vi "Testing (not part of comp).vi"() -> ()   [LabVIEW 2013]
panel:
  in  "Down":bool
  in  "Up":bool
  in  "ON/OFF":bool
  in  "Return":bool
  in  "stop":bool
  in  "4 ft":bool
  # "Pickup"
  # "LED"
  # "Shooter"
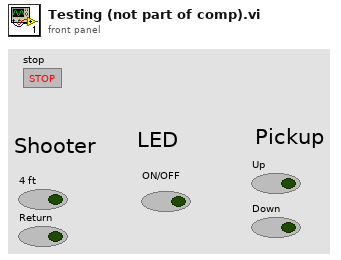
[diagram p1: front panel]
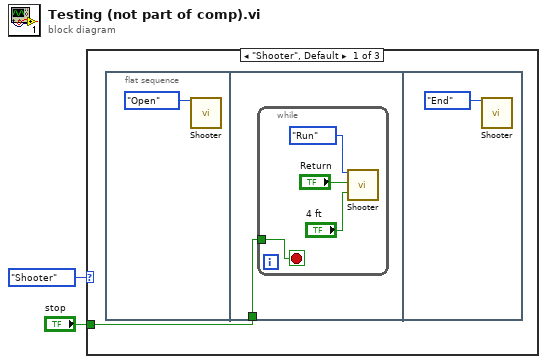
[diagram p0: block diagram]
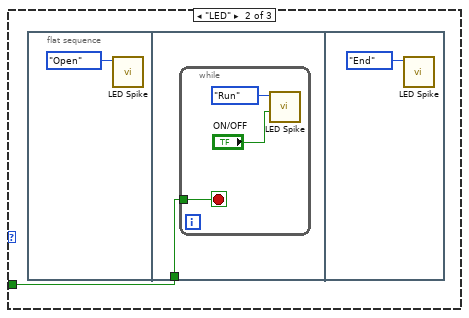
[diagram p2: hidden frame]
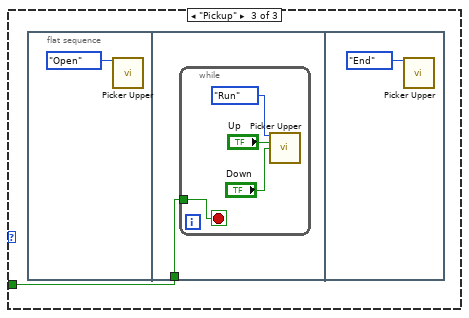
[diagram p3: hidden frame]
diagram:
  n1 = case shown="\"Shooter\", Default" enum16{"Shooter", "LED", "Pickup"}."Shooter" ("Enum") {
    tunnel: "stop" -> [w3 w11 w18]
    frame "Shooter", Default {
      n2 = flat-sequence {
        tunnel: w3 -> [w5]
        frame #0 {
          n3 = call "Shooter.vi"("State Control"=enum16{"Open", "Run", "End"}."Open") -> ()  [unwired: 17 in, 2 out]
        }
        frame #1 {
          n4 = while {
            tunnel: w5 -> [w7]
            stop <- w7 stop-if-true
            n5 = call "Shooter.vi"("State Control"=enum16{"Open", "Run", "End"}."Run", "Return"="Return", "4 ft"="4 ft") -> ()  [unwired: 15 in, 2 out]
          }
        }
        frame #2 {
          n6 = call "Shooter.vi"("State Control"=enum16{"Open", "Run", "End"}."End") -> ()  [unwired: 17 in, 2 out]
        }
      }
    }
    frame "LED" {
      n7 = flat-sequence {
        tunnel: w11 -> [w13]
        frame #0 {
          n8 = call "LED Spike.vi"("State"=enum16{"Open", "Run", "End"}."Open" ("State Control")) -> ()  [unwired: 11 in]
        }
        frame #1 {
          n9 = while {
            tunnel: w13 -> [w16]
            stop <- w16 stop-if-true
            n10 = call "LED Spike.vi"("ON/OFF"="ON/OFF", "State"=enum16{"Open", "Run", "End"}."Run" ("State Control")) -> ()  [unwired: 10 in]
          }
        }
        frame #2 {
          n11 = call "LED Spike.vi"("State"=enum16{"Open", "Run", "End"}."End" ("State Control")) -> ()  [unwired: 11 in]
        }
      }
    }
    frame "Pickup" {
      n12 = flat-sequence {
        tunnel: w18 -> [w20]
        frame #0 {
          n13 = call "Picker Upper.vi"("State Control"=enum16{"Open", "Run", "End"}."Open") -> ()  [unwired: 13 in, 2 out]
        }
        frame #1 {
          n14 = while {
            tunnel: w20 -> [w24]
            stop <- w24 stop-if-true
            n15 = call "Picker Upper.vi"("State Control"=enum16{"Open", "Run", "End"}."Run", "Up"="Up", "Down"="Down") -> ()  [unwired: 11 in, 2 out]
          }
        }
        frame #2 {
          n16 = call "Picker Upper.vi"("State Control"=enum16{"Open", "Run", "End"}."End") -> ()  [unwired: 13 in, 2 out]
        }
      }
    }
  }
